vi "SetOnOffTemp.vi"(1 "Error In":errorcluster, 2 "Boolean":bool) -> (0 "Error Out":errorcluster)   [LabVIEW 2014]
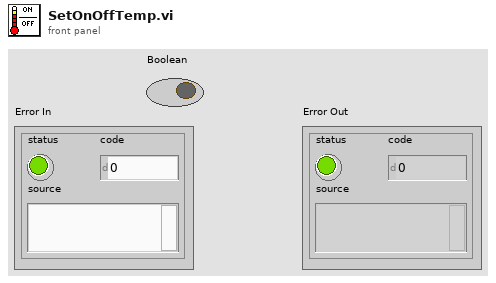
[diagram p1: front panel]
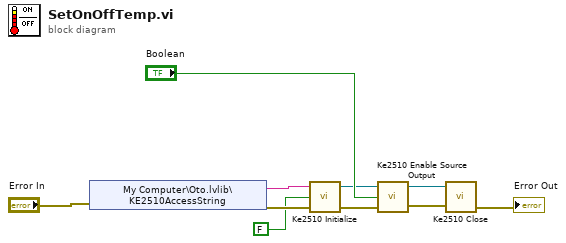
[diagram p0: block diagram]
diagram:
  n1 = shared-variable "My Computer\\Oto.lvlib\\KE2510AccessString"(error in="Error In") -> (w4:string, error out=w9:errorcluster)
  n2 = call <instrlib>:"Ke2510 Initialize.vi"("error in (no error)"=w9, "reset device"=FALSE, "resource name"=w4) -> ("error out"=w8:errorcluster, "instrument handle"=w3:refnum<visa-resource-name>)  [unwired: 1 out]
  n3 = call <instrlib>:"Ke2510 Enable Source Output.vi"("error in (no error)"=w8, "enabled"="Boolean", "instrument handle"=w3) -> ("error out"=w7:errorcluster, "instrument handle out"=w2:refnum<visa-resource-name>)  [unwired: 1 out]
  n4 = call <instrlib>:"Ke2510 Close.vi"("instrument handle"=w2, "error in (no error)"=w7) -> ("error out"=→"Error Out":errorcluster)  [unwired: 1 in, 1 out]
